vi "Find Owned Test Methods in Test Case.vi"(8 "error in (no error)":errorcluster, 10 "Test Case Class Path":path, 11 "Test Finder In":refnum<class "Test Finder.lvclass">) -> (0 "error out":errorcluster, 2 "Test Methods Out":map{string, path}(c390), 3 "Test Finder Out":refnum<class "Test Finder.lvclass">)   [LabVIEW 2020, in "Test Finder.lvclass"]
uses:
  Test Finder.lvclass
  Test Finder.lvclass/Test Finder.ctl
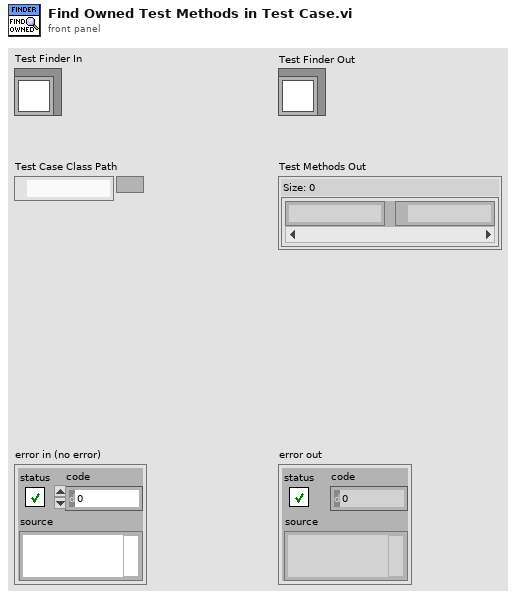
[diagram p1: front panel]
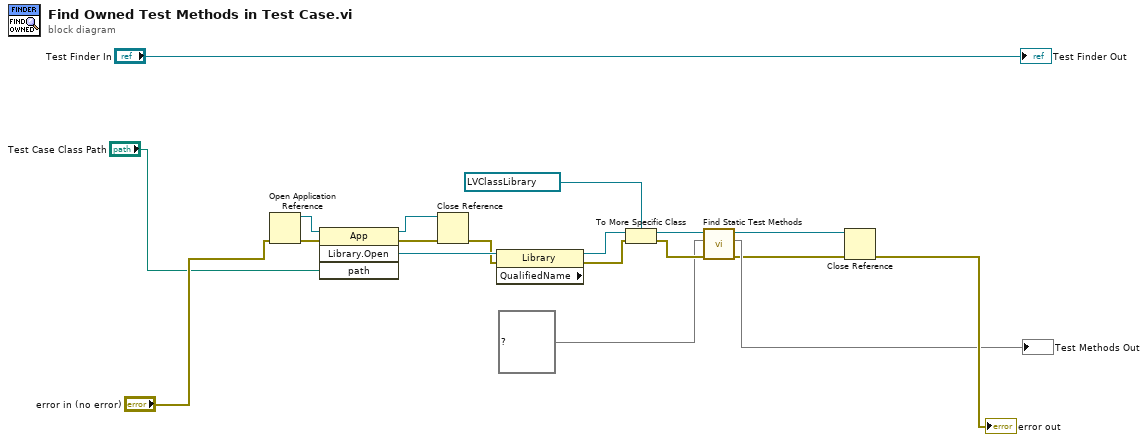
[diagram p0: block diagram]
diagram:
  n1 = Open Application Reference(8:"error in (no error)") -> (0:w18:errorcluster, 3:w19:refnum<vi>)  [unwired: 3 in]
  n2 = invoke on="Invoke Node" class="App" method="Library.Open"(reference=w19, error in=w18, "path"="Test Case Class Path") -> (reference out=w16:refnum<vi>, error out=w17:errorcluster, "Open Library"=w7:refnum<vi>)  [unwired: 1 in, 1 out]
  n3 = Close Reference(reference=w16, error in (no error)=w17) -> (error out=w5:errorcluster)
  n4 = property on="Property Node" class="Library" props=["QualifiedName"](reference=w7, error in=w5) -> (reference out=w6:refnum<vi>, error out=w4:errorcluster)  [unwired: 1 out]
  n5 = To More Specific Class(target class=refnum<vi> refnum ("Library:Open"), reference=w6, error in=w4) -> (specific class reference=w13:refnum<vi>, error out=w11:errorcluster)
  n6 = call "Find Static Test Methods.vi"("error in (no error)"=w11, "Test Methods In"=map{string, path} {}, "LVClassLibrary in"=w13) -> ("error out"=w9:errorcluster, "Test Methods Out"=→"Test Methods Out":map{string, path}, "LVClassLibrary out"=w12:refnum<vi>)  [unwired: 6 in]
  n7 = Close Reference(reference=w12, error in (no error)=w9) -> (error out=→"error out":errorcluster)
  "Test Finder Out" <- "Test Finder In"
